vi "SortRefs.vi"(8 "error in":errorcluster, 11 "Refs In":refnum<k20>[](array[refnum])) -> (0 "error out":errorcluster, 3 "Refs Out":refnum<k20>[](array[refnum]))   [LabVIEW 2011]
uses:
  Program Files/National Instruments/LabVIEW 2011/resource/objmgr/nisysapi.rc
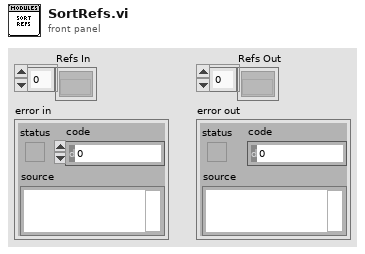
[diagram p1: front panel]
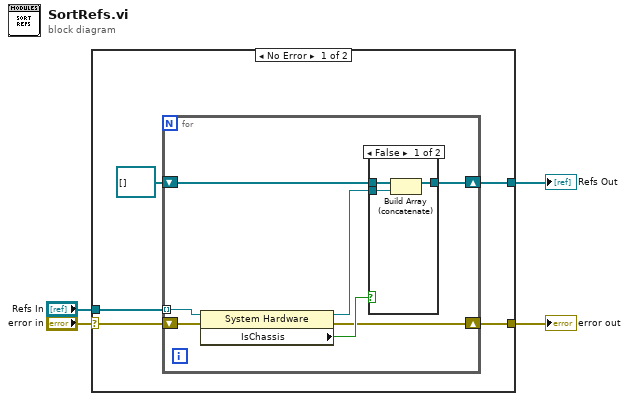
[diagram p0: block diagram]
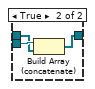
[diagram p2: hidden frame]
diagram:
  n1 = case shown="No Error" "error in" {
    selector: "error in" -> [w5 w23]
    tunnel: "Refs In" -> [w9 _]
    tunnel: [w8 _] -> w3
    tunnel: [w6 w23] -> w2
    frame No Error {
      n2 = for {
        tunnel: w9 -> [w16] mode=indexing
        shift-right: [w13] -> w8
        shift-left: refnum<k20>[] [] -> [w14]
        shift-right: [w11] -> w6
        shift-left: w5 -> [w10]
        n3 = property class="System Hardware"(reference=w16, error in=w10) -> (reference out=w15:refnum<k20>, error out=w11:errorcluster, "IsChassis"=w12:bool)
        n4 = case shown="False" w12 {
          tunnel: w15 -> [w18 w22]
          tunnel: w14 -> [w19 w21]
          tunnel: [w17 w20] -> w13
          frame False {
            n5 = Build Array (concatenate)(w19, w18) -> (w17:refnum<k20>[])
          }
          frame True {
            n6 = Build Array (concatenate)(w22, w21) -> (w20:refnum<k20>[])
          }
        }
      }
    }
    frame Error {
    }
  }
  "Refs Out" <- w3
  "error out" <- w2
